vi "tetragon extraction.vi"(7 "Options":T2={"Interpolation Type"=enum."Bilinear", "Destination Width"=497, "Destination Height"=299, "Fill Value"=100.0}, 8 "error in (no error)":errorcluster, 9 "Image Type":T1 items=["Grayscale (U8)", "Grayscale (I16)", "Grayscale (SGL)", "Complex (CSG)", "RGB (U32)", "HSL (U32)", "RGB (U64)", "Grayscale (U16)"], 10 "target img":u16[][](array[numeric])=array300x498[149400 elements], 11 "X":dbl[](array[numeric])=[-7.233324409925488, -9.973293657815278, 492.1177782221989, 7.125974863451136, 476.09973407077223, 286.0595696636521, 12.284589284003047, 315.85020829622647]) -> (0 "error out":errorcluster, 2 "Image Pixels (U16)":u16[][](array[numeric]), 3 "Image Pixels (U8)":u8[][](array[numeric]))   [LabVIEW 2024]
uses:
  <vilib>/vision/NI_Vision_Development_Module.lvlib
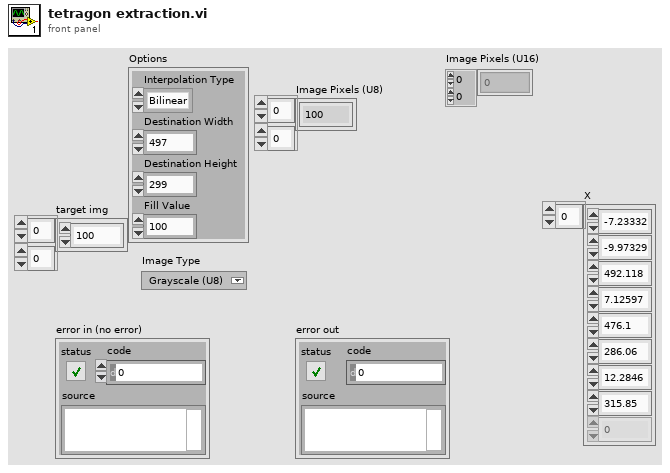
[diagram p1: front panel]
types:
  T1 = typedef "Image Type" = u32
  T2 = cluster{"Interpolation Type":enum32{"Zero Order", "Bilinear", "Quadratic", "Cubic", "Bilinear Fixed"}, "Destination Width":u32, "Destination Height":u32, "Fill Value":sgl}
  T3 = typedef "IMAQ Image.ctl" = refnum<image>
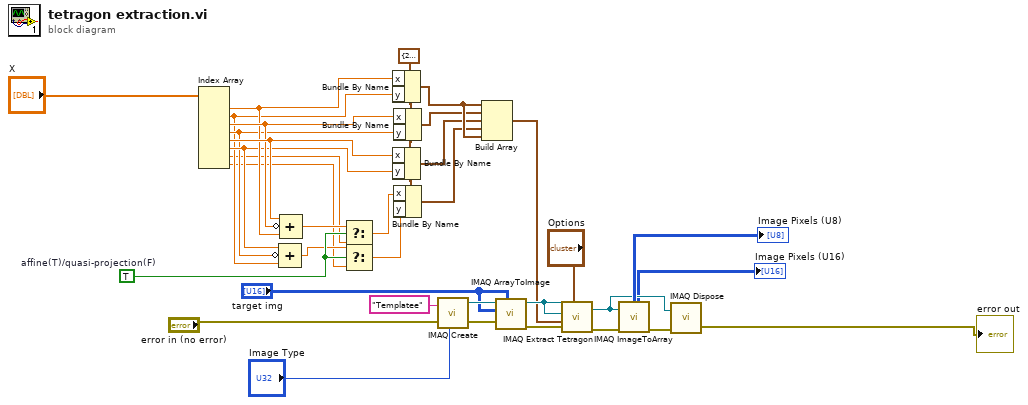
[diagram p0: block diagram]
diagram:
  w9 = TRUE  # affine(T)/quasi-projection(F)
  w21 = cluster{"x":sgl, "y":sgl} {"x"=220.0, "y"=100.0} ("Position 2")
  n1 = Index Array(array="X") -> (element #1=w13:dbl, element #2=w10:dbl, element #3=w14:dbl, element #4=w11:dbl, element #5=w15:dbl, element #6=w12:dbl, element #7=w6:dbl, element #8=w5:dbl)  [unwired: 8 in]
  n2 = Compound Arithmetic op=ADD(w12, invert w11, w10) -> (w7:dbl)
  n3 = Compound Arithmetic op=ADD(w15, invert w14, w13) -> (w8:dbl)
  n4 = Select(t=w8, s=w9, f=w6) -> (s? t:f=w4:dbl)
  n5 = Select(t=w7, s=w9, f=w5) -> (s? t:f=w3:dbl)
  n6 = Bundle By Name(cluster=w21, "x"=w13, "y"=w10) -> (w25:cluster{"x":sgl, "y":sgl})
  n7 = Bundle By Name(cluster=w21, "x"=w15, "y"=w12) -> (w23:cluster{"x":sgl, "y":sgl})
  n8 = Bundle By Name(cluster=w21, "x"=w14, "y"=w11) -> (w22:cluster{"x":sgl, "y":sgl})
  n9 = Bundle By Name(cluster=w21, "x"=w4, "y"=w3) -> (w24:cluster{"x":sgl, "y":sgl})
  n10 = call "IMAQ Create"("Image Name"="Templatee", "Image Type"="Image Type", "error in (no error)"="error in (no error)") -> ("New Image"=w28:T3, "error out"=w29:errorcluster)  [unwired: 2 in]
  n11 = Build Array(w25, w22, w23, w24, w25) -> (w17:cluster{"x":sgl, "y":sgl}[])
  n12 = call "IMAQ ArrayToImage"("Image Pixels (U16)"="target img", "error in (no error)"=w29, "Image Pixels (U8)"="target img", "Image"=w28) -> ("error out"=w30:errorcluster, "Image Out"=w19:T3)  [unwired: 6 in]
  n13 = call-poly "IMAQ Extract Tetragon"("Options"="Options", "error in (no error)"=w30, "Tetragon"=w17, "Image Dst"=w19, "Image Src"=w19) -> ("error out"=w31:errorcluster, "Image Dst Out"=w32:T3)  [unwired: 5 in]
  n14 = call "IMAQ ImageToArray"("error in (no error)"=w31, "Image"=w32) -> ("Image Pixels (U16)"=→"Image Pixels (U16)":u16[][], "error out"=w18:errorcluster, "Image Pixels (U8)"=→"Image Pixels (U8)":u8[][])  [unwired: 2 in, 2 out]
  n15 = call "IMAQ Dispose"("Image"=w32, "error in (no error)"=w18) -> ("error out"=→"error out":errorcluster)  [unwired: 4 in]
